vi "Live_Plot.vi"() -> ()   [LabVIEW 2013]
uses:
  <userlib>/Accelerator/User Interface/Controls/Graph.ctl
  <userlib>/Accelerator/User Interface/Controls/Constraints.ctl
  <userlib>/Accelerator/User Interface/Controls/Waveforms.ctl
  <vilib>/Utility/miscctls.llb/LVPointTypeDef.ctl
  <userlib>/_OpenG.lib/comparison/comparison.llb/Variant Changed__ogtk.vi
  <userlib>/_OpenG.lib/array/array.llb/Empty 1D Array (Variant)__ogtk.vi
panel:
  out "Multipliers":dbl[](array[numeric])
  out "Cursor grabbed?":bool
  out "Month":dbl
  out "Updating...":bool
  out "Density (g/cc)":dbl=7.874000072479248 min=0.0 max=25.0
  in  "Tab Control":T1(tab)
  out "Number of Matching Events:":i64
  out "Percent of triggers that fit constraints:":dbl format="%#_4g%"
  out "Total Number of triggers:":i64
  in  "Enable\nTimestamp":bool
  out "Constrained Distribution":T2
  in  "Save Image":bool
  in  "Constraints":T3={"Upper Timestamp Range"=timestamp(0 s since 1904-01-01), "Lower Timestamp Range"=timestamp(0 s since 1904-01-01), "Experiment Group:"="", "Experiment Name:"=[], "Upper Velocity Limit (km/s)"=0.0, "Lower Velocity Limit (km/s)"=0.0, "Upper Mass Limit (kg)"=0.0, "Lower Mass Limit (kg)"=0.0, "name array"=[], "Estimate Quality"={0.0, 5.0}} {"Estimate Quality" scale=0.0..5.0; "Lower Mass Limit (kg)" min=0.0 step=1e-20; "Upper Mass Limit (kg)" min=0.0 step=1e-20}
  in  "Velocity":dbl=1.0 min=0.1 max=100.0
  in  "Mass":dbl=2.638602750087072e-13 min=1e-20 max=1e-10
  in  "Radius (µm)":dbl=2.0 min=0.00671912 max=14.4759
  in  "Reset Visible Time":bool caption="Save Metadata"
  in  "Time Visible":dbl=5000.0 min=0.0 step=1000.0
  out "Selected Waveforms":u64[](array[numeric])
  out "Waveforms":T4[](array[typedef])
  out "Max Time":dbl=5000.0
  in  "If this was the big acc...":bool
  out "Max Query Time":dbl
  in  "Pelletron Voltage (MV):":dbl=2.0
  out "Experiment Start":timestamp
  out "Test":bool caption="Test Database in use:"
  out "Test 2":bool caption="Production Database in use:"
  in  "error in (no error)":errorcluster
  out "error out":errorcluster
  in  "Vnoise Estimate:":dbl=0.005
  in  "Sensitivity:":dbl=12100000000000.0
  in  "Update interval (s)":dbl=5.0 min=1.0 max=60.0 step=1.0 format="%#_4g"
  out "Query Time":dbl
  in  "Small?":bool
  in  "Clear Errors":bool
  in  "Exit":bool
  # "Live Plot of Current Experiment"
  # "Cursor"
  # "Plot Settings:"
  # "ODBC Connection Status:"
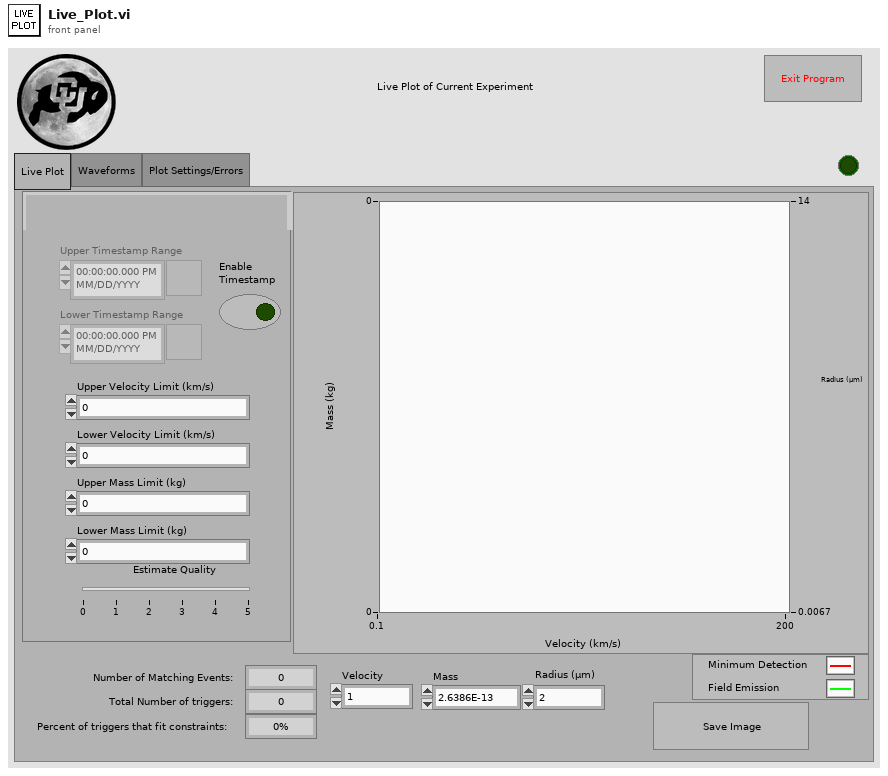
[diagram p1: front panel]
types:
  T1 = enum32{"Live Plot", "Waveforms", "Plot Settings/Errors"}
  T2 = typedef "Graph.ctl" = cluster{cluster{"Vnoise":dbl, "Vnoise":dbl}[]}[]
  T3 = typedef "Constraints.ctl" = cluster{"Upper Timestamp Range":timestamp, "Lower Timestamp Range":timestamp, "Experiment Group:":string, "Experiment Name:":i32[], "Upper Velocity Limit (km/s)":dbl, "Lower Velocity Limit (km/s)":dbl, "Upper Mass Limit (kg)":dbl, "Lower Mass Limit (kg)":dbl, "name array":string[], "Estimate Quality":cluster{dbl, dbl}}
  T4 = typedef "Waveforms.ctl" = cluster{"id_dust_event":u64, "Time Stamp":timestamp, "Velocity":dbl, "Mass":dbl, "Charge":dbl, "Radius":dbl, "Waveform Graph":sgl[][], "Quality":i32}
  T5 = typedef "LVPointTypeDef.ctl" = cluster{"Horizontal":i16, "Vertical":i16}
  T6 = typedef "LVRectTypeDef.ctl" = cluster{"Left":i16, "Top":i16, "Right":i16, "Bottom":i16}
  T7 = enum8{"Enabled", "Disabled", "Disabled and Grayed Out"}
  T8 = typedef "DisplayExperimentSetting.ctl" = cluster{"Current Experiment Name:":string, "Current Experiment Description:":string, "Current Experiment Group ID:":string, "Experiment Settings Last Updated At:":timestamp}
  T9 = typedef "Query_Dust_Event.ctl" = cluster{"Dust Event ID":i64, "Integer Timestamp":i64, "Velocity":dbl, "Mass":dbl, "Charge":sgl, "Radius":sgl, "Passed_3rd_Detector":i8, "High Voltage":sgl, "+ High Voltage Supply":sgl, "- High Voltage Supply":sgl, "HV Control Difference":sgl, "Vacuum Pressure":sgl, "Radiation":sgl, "Column Current":sgl, "Lost Charge":sgl, "Chain Current":sgl, "Control High Voltage":sgl, "Current Group Name:":string, "Current Experiment Name:":string, "Current Experiment Description:":string, "Estimate Source":T10, "Estimate Quality":i8, "File Location":T11, "Dust Type":string, "Dust Density":sgl}
  T10 = typedef "Estimate_source.ctl" = i8
  T11 = typedef "File_location.ctl" = i8
  T12 = typedef "imagedata.ctl" = cluster{"image type":i32, "image depth":i32, "image":u8[], "mask":u8[], "colors":u32[], "Rectangle":cluster{"left":i16, "top":i16, "right":i16, "bottom":i16}}
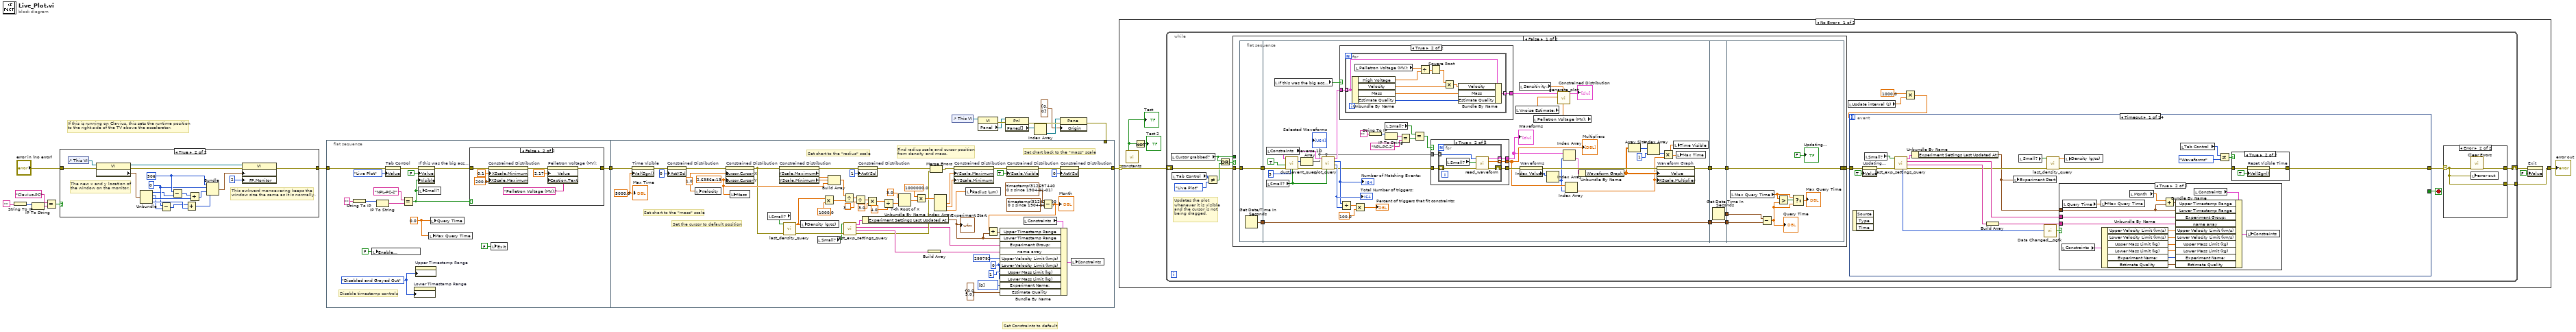
[diagram p0: block diagram]
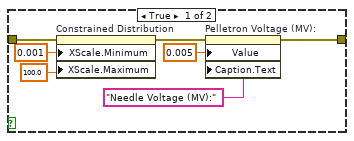
[diagram p3: hidden frame]
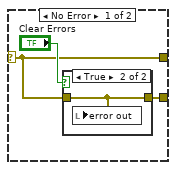
[diagram p4: hidden frame]
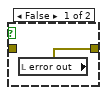
[diagram p5: hidden frame]
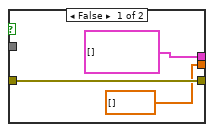
[diagram p6: hidden frame]
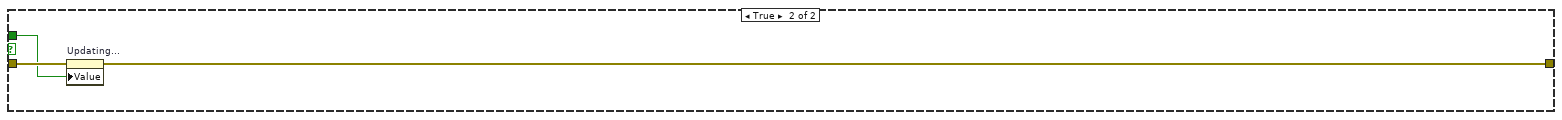
[diagram p8: hidden frame]
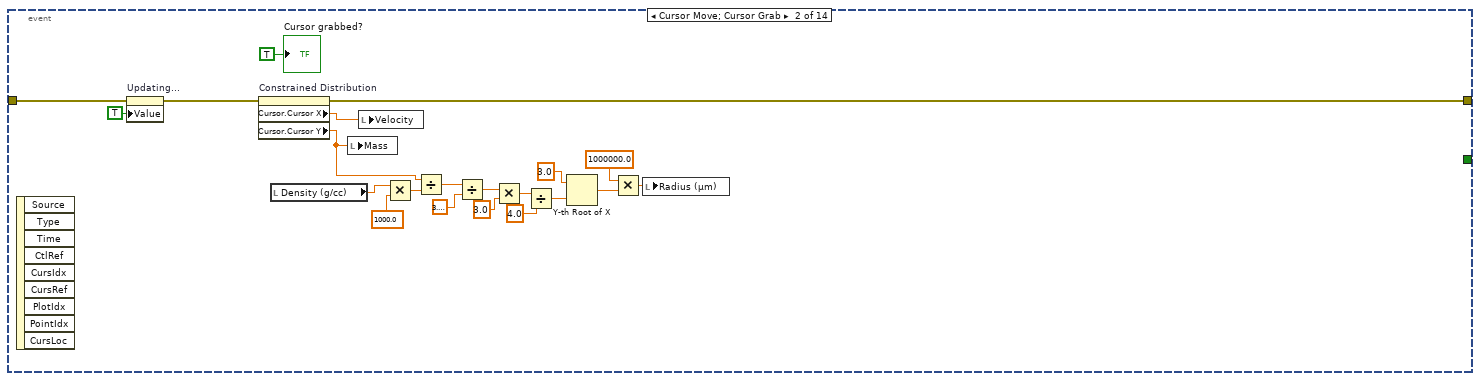
[diagram p11: hidden frame]
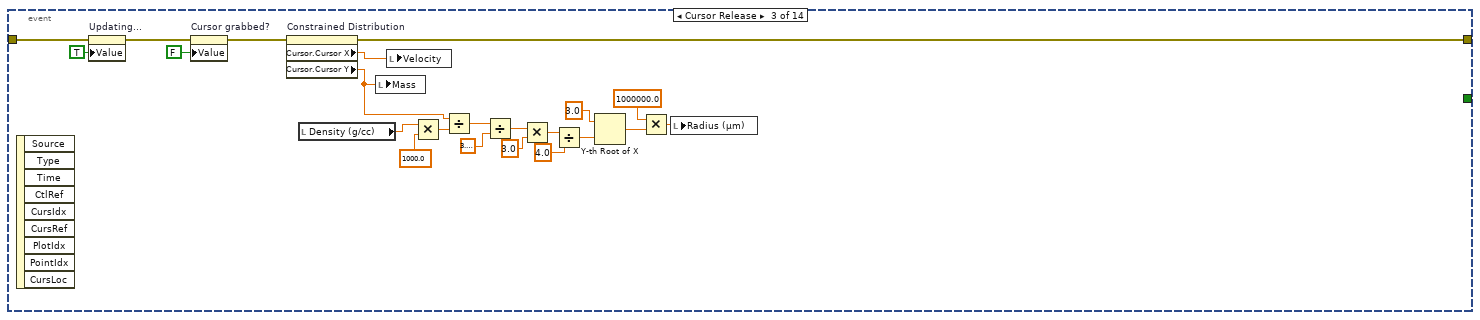
[diagram p12: hidden frame]
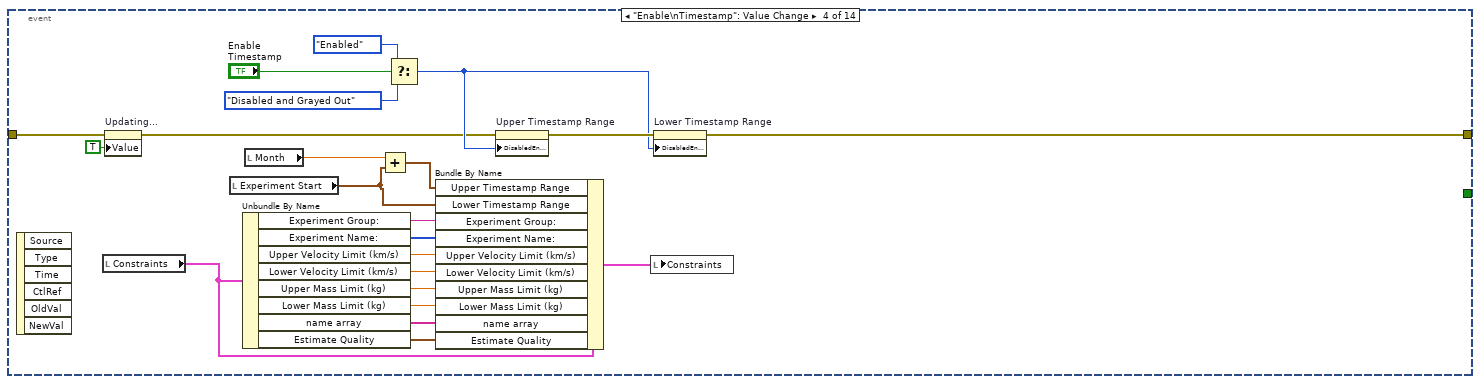
[diagram p13: hidden frame]
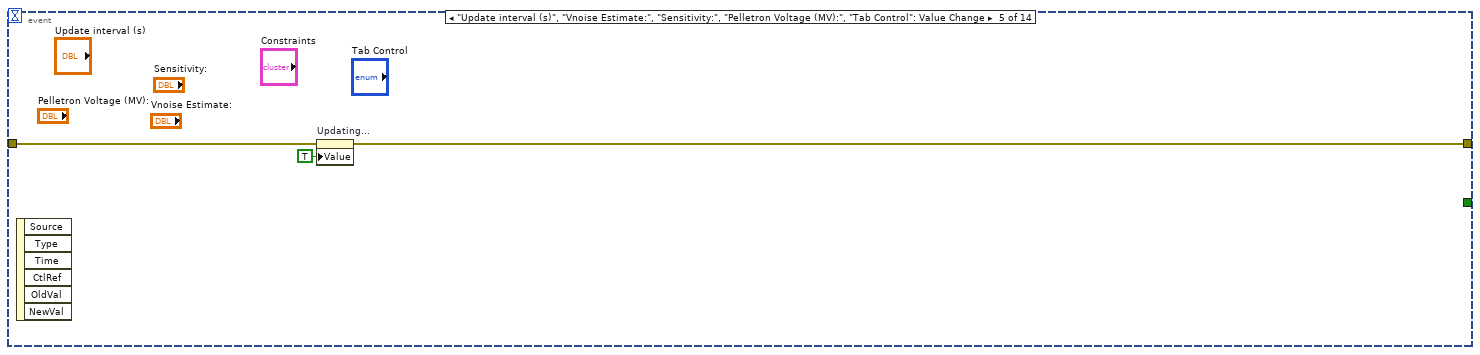
[diagram p14: hidden frame]
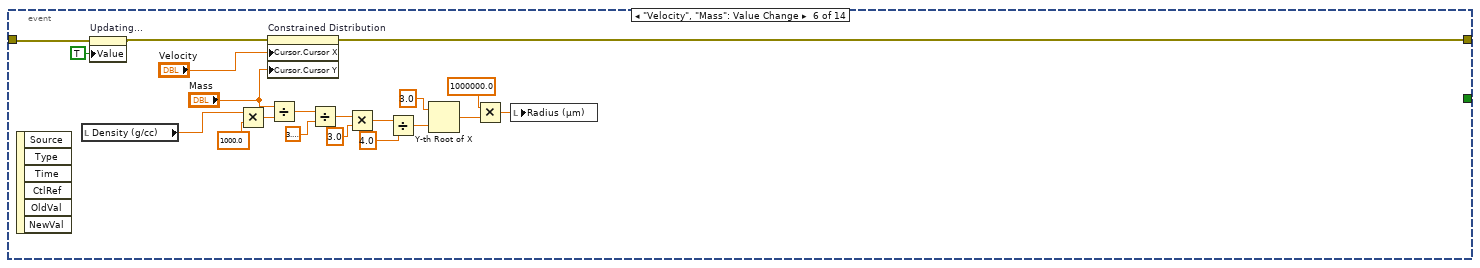
[diagram p15: hidden frame]
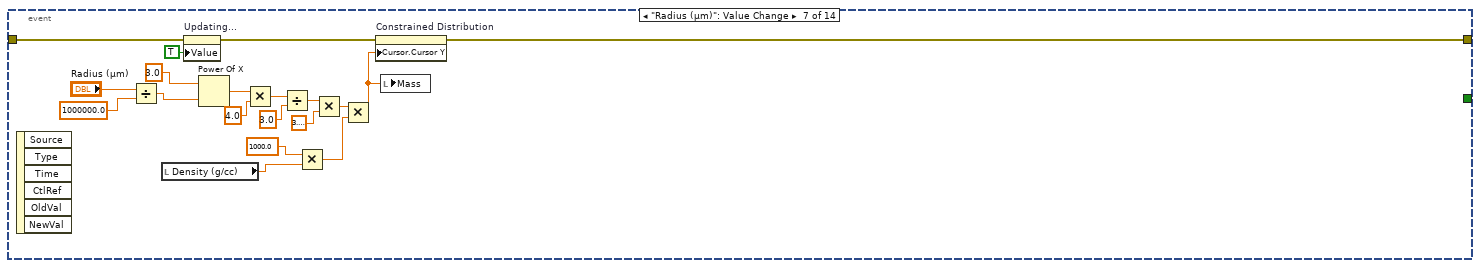
[diagram p16: hidden frame]
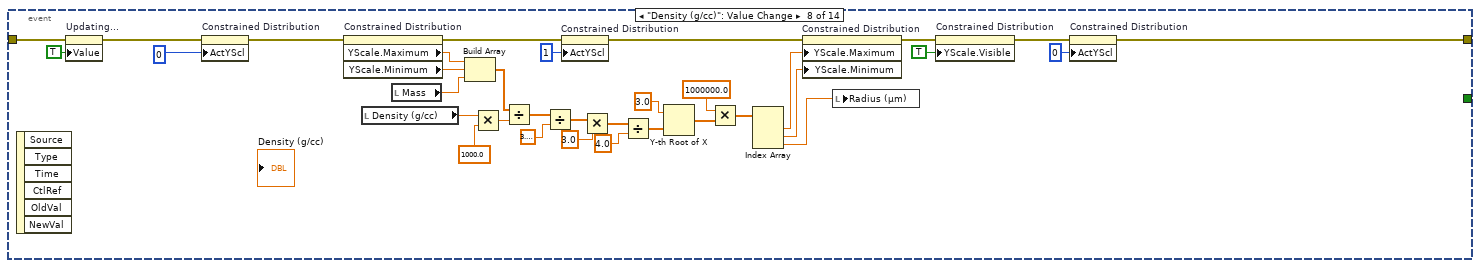
[diagram p17: hidden frame]
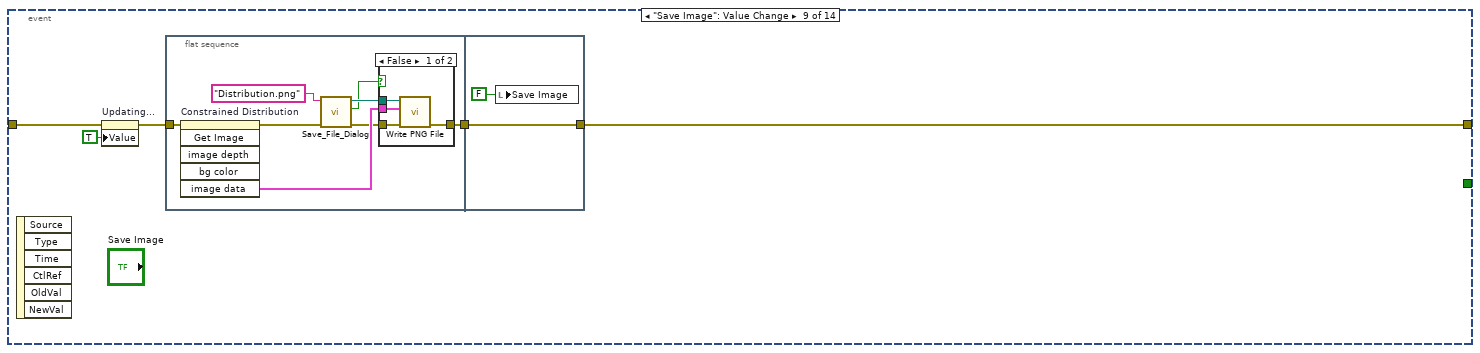
[diagram p18: hidden frame]
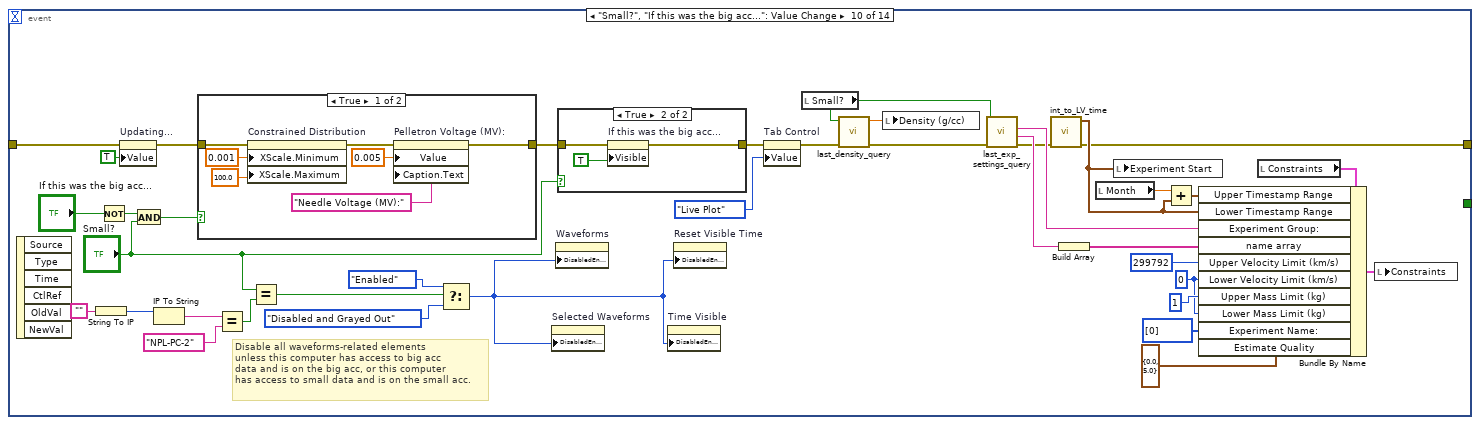
[diagram p20: hidden frame]
diagram:
  # "If this is running on Clavius, this sets the runtime position\nto the right side of the TV above the accelerator."
  # "Set Constraints to default"
  n1 = String To IP(1:"" ("name")) -> (0:w5:u32)
  n2 = IP To String(2:w5) -> (0:w3:string)  [unwired: 1 in]
  n3 = Equal?(x="Clavius-PC", y=w3) -> (x = y?=w7:bool)
  n4 = case shown="True" w7 {
    tunnel: "error in (no error)" -> [w19 w22]
    tunnel: [w19 w20] -> w1
    frame False {
    }
    frame True {
      w27 = i16 0 ("Top")
      w28 = i16 506 ("Left")
      # "This awkward manoevering keeps the\nwindow size the same as it is normally."
      # "The new x and y location of\nthe window on the monitor."
      n5 = control-ref of="This VI"() -> (w36:refnum<vi>)
      n6 = property class="VI"(reference=w36, error in=w22) -> (reference out=w32:refnum<vi>, error out=w21:errorcluster, "Front Panel.WinBounds"=w31:T6)
      n7 = Unbundle(w31) -> ("Left"=w26:i16, "Top"=w25:i16, "Right"=w30:i16, "Bottom"=w29:i16)
      n8 = Subtract(x=w27, y=w25) -> (x-y=w24:i16)
      n9 = Subtract(x=w28, y=w26) -> (x-y=w23:i16)
      n10 = Add(x=w24, y=w29) -> (x+y=w33:i16)
      n11 = Add(x=w23, y=w30) -> (x+y=w34:i16)
      n12 = Bundle("Left"=w28, "Top"=w27, w34, w33) -> (w37:cluster{"Left":i16, "Top":i16, i16, i16})  [unwired: 1 in]
      n13 = property class="VI"(reference=w32, error in=w21, "Front Panel.WinBounds"=w37, "FP.Monitor"=u16 2 ("Front Panel Window:Monitor")) -> (error out=w20:errorcluster)  [unwired: 1 out]
    }
  }
  n14 = flat-sequence {
    tunnel: [w48] -> w8
    tunnel: w1 -> [w40]
    tunnel: [w123] -> w10
    tunnel: w9 -> [_]
    tunnel: w8 -> [w73]
    frame #0 {
      w41 = 0.0 ("Query Time")
      w45 = T7."Disabled and Grayed Out" ("Disabled")
      # "Disable timestamp controls"
      n15 = String To IP(1:"" ("name")) -> (0:w51:u32)
      n16 = local write "Enable\nTimestamp"(FALSE ("Enable\nTimestamp")) -> ()
      n17 = IP To String(2:w51) -> (0:w49:string)  [unwired: 1 in]
      n18 = property on="Tab Control" class="TabCtl (strict)"(error in=w40, "Value"=T1."Live Plot" ("Tab Control")) -> (error out=w39:errorcluster)  [unwired: 1 in, 1 out]
      n19 = Equal?(x="NPL-PC-2", y=w49) -> (x = y?=w42:bool)
      n20 = property on="Lower Timestamp Range" class="AbsTime (strict)"("DisabledEnum"=w45) -> ()  [unwired: 2 in, 2 out]
      n21 = property on="Upper Timestamp Range" class="AbsTime (strict)"("DisabledEnum"=w45) -> ()  [unwired: 2 in, 2 out]
      n22 = property on="If this was the big acc..." class="Bool (strict)"(error in=w39, "Value"=FALSE ("If this was the big acc..."), "Visible"=w42) -> (error out=w44:errorcluster)  [unwired: 1 in, 1 out]
      n23 = local write "Small?"(w42) -> ()
      n24 = local write "Max Query Time"(w41) -> ()
      n25 = local write "Query Time"(w41) -> ()
      n26 = case shown="False" w42 {
        tunnel: [w57 w64] -> w48
        tunnel: w44 -> [w54 w61]
        frame True {
          n27 = property on="Constrained Distribution" class="XYGraph (strict)"(error in=w54, "XScale.Minimum"=0.001 ("X Scale.Range:Minimum"), "XScale.Maximum"=100.0 ("X Scale.Range:Maximum")) -> (error out=w53:errorcluster)  [unwired: 1 in, 1 out]
          n28 = property on="Pelletron Voltage (MV):" class="DigNum (strict)"(error in=w53, "Value"=0.005 ("Pelletron Voltage (MV):"), "Caption.Text"="Needle Voltage (MV):") -> (error out=w57:errorcluster)  [unwired: 1 in, 1 out]
        }
        frame False {
          n29 = property on="Constrained Distribution" class="XYGraph (strict)"(error in=w61, "XScale.Minimum"=0.1 ("X Scale.Range:Minimum"), "XScale.Maximum"=200.0 ("X Scale.Range:Maximum")) -> (error out=w60:errorcluster)  [unwired: 1 in, 1 out]
          n30 = property on="Pelletron Voltage (MV):" class="DigNum (strict)"(error in=w60, "Value"=2.17 ("Pelletron Voltage (MV):"), "Caption.Text"="Pelletron Voltage (MV):") -> (error out=w64:errorcluster)  [unwired: 1 in, 1 out]
        }
      }
      n31 = local write "Exit"(FALSE ("Exit")) -> ()
    }
    frame #1 {
      w71 = 5000.0 ("Max Time")
      w122 = 2.6386e-13 ("Mass")
      w109 = 1.0 ("Velocity")
      w115 = 0
      # "Set chart back to the \"mass\" scale"
      # "Set chart to the \"radius\" scale"
      # "Set chart to the \"mass\" scale"
      # "Find radius scale and cursor position\nfrom density and mass."
      # "Set the cursor to default position"
      n32 = property on="Time Visible" class="DigNum (strict)"(error in=w73, "Val(Sgnl)"=w71) -> (error out=w72:errorcluster)  [unwired: 1 in, 1 out]
      n33 = property on="Constrained Distribution" class="XYGraph (strict)"(error in=w72, "ActYScl"=0 ("Active Y Scale")) -> (error out=w78:errorcluster)  [unwired: 1 in, 1 out]
      n34 = local write "Velocity"(w109) -> ()
      n35 = property on="Constrained Distribution" class="XYGraph (strict)"(error in=w78, "Cursor.Cursor X"=w109, "Cursor.Cursor Y"=w122) -> (error out=w80:errorcluster)  [unwired: 1 in, 1 out]
      n36 = local write "Mass"(w122) -> ()
      n37 = local read "Small?"() -> (w77:bool)
      n38 = property on="Constrained Distribution" class="XYGraph (strict)"(error in=w80) -> (error out=w96:errorcluster, "YScale.Maximum"=w95:dbl, "YScale.Minimum"=w94:dbl)  [unwired: 1 in, 1 out]
      n39 = call <userlib>:"last_density_query.vi"("error in (no error)"=w80, "Small?"=w77) -> ("error out"=w82:errorcluster, "Density"=w81:dbl)  [unwired: 8 in]
      n40 = local write "Density (g/cc)"(w81) -> ()
      n41 = local read "Small?"() -> (w76:bool)
      n42 = Multiply(x=w81, y=1000.0) -> (x*y=w100:dbl)
      n43 = Build Array(w95, w94, w122) -> (w93:dbl[])
      n44 = Divide(x=w93, y=w100) -> (x/y=w108:dbl[])
      n45 = call <userlib>:"last_exp_settings_query.vi"("error in (no error)"=w82, "Small?"=w76) -> ("error out"=w70:errorcluster, "Experiment Name"=w110:string, "Group Name"=w67:string, "Experiment Settings"=w69:T8)  [unwired: 4 in, 2 out]
      n46 = Divide(x=w108, y=3.141592653589793) -> (x/y=w106:dbl[])
      n47 = property on="Constrained Distribution" class="XYGraph (strict)"(error in=w96, "ActYScl"=1 ("Active Y Scale")) -> (error out=w92:errorcluster)  [unwired: 1 in, 1 out]
      n48 = Unbundle By Name(w69) -> ("Experiment Settings Last Updated At:"=w68:timestamp)
      "Experiment Start" <- w68
      n49 = Multiply(x=w106, y=3.0) -> (x*y=w104:dbl[])
      n50 = Divide(x=w104, y=4.0) -> (x/y=w102:dbl[])
      n51 = Y-th Root of X(1:w102, 2:3.0 ("y")) -> (0:w98:dbl[])
      n52 = Multiply(x=1000000.0, y=w98) -> (x*y=w90:dbl[])
      n53 = Build Array(w110) -> (w74:string[])
      n54 = Merge Errors(w92, w70) -> (w75:errorcluster)
      n55 = Index Array(array=w90) -> (element #1=w88:dbl, element #2=w87:dbl, element #3=w86:dbl)  [unwired: 3 in]
      n56 = property on="Constrained Distribution" class="XYGraph (strict)"(error in=w75, "YScale.Maximum"=w88, "YScale.Minimum"=w87) -> (error out=w89:errorcluster)  [unwired: 1 in, 1 out]
      n57 = local write "Radius (µm)"(w86) -> ()
      n58 = property on="Constrained Distribution" class="XYGraph (strict)"(error in=w89, "YScale.Visible"=TRUE ("Y Scale.Visible")) -> (error out=w84:errorcluster)  [unwired: 1 in, 1 out]
      n59 = local read "Constraints"() -> (w121:T3)
      n60 = Subtract(x=timestamp(3126974400 s since 1904-01-01) ("current time"), y=timestamp(3124296000 s since 1904-01-01) ("current time")) -> (x-y=w118:dbl)
      "Month" <- w118
      n61 = Add(x=w118, y=w68) -> (x+y=w119:timestamp)
      n62 = Bundle By Name(cluster=w121, "Upper Timestamp Range"=w119, "Lower Timestamp Range"=w68, "Experiment Group:"=w67, "name array"=w74, "Upper Velocity Limit (km/s)"=299792, "Lower Velocity Limit (km/s)"=w115, "Upper Mass Limit (kg)"=1, "Lower Mass Limit (kg)"=w115, "Experiment Name:"=i32[] [0], "Estimate Quality"=cluster{dbl, dbl} {0.0, 5.0}) -> (w120:T3)
      n63 = property on="Constrained Distribution" class="XYGraph (strict)"(error in=w84, "ActYScl"=0 ("Active Y Scale")) -> (error out=w123:errorcluster)  [unwired: 1 in, 1 out]
      n64 = local write "Constraints"(w120) -> ()
      "Max Time" <- w71
    }
  }
  n65 = control-ref of="This VI"() -> (w17:refnum<vi>)
  n66 = property class="VI"(reference=w17) -> (error out=w16:errorcluster, "Panel"=w15:refnum<vi>)  [unwired: 1 in, 1 out]
  n67 = property class="Pnl"(reference=w15, error in=w16) -> (error out=w14:errorcluster, "Panes[]"=w13:refnum<vi>[])  [unwired: 1 out]
  n68 = Index Array(array=w13) -> (element=w12:refnum<vi>)  [unwired: 1 in]
  n69 = property class="Pane"(reference=w12, error in=w14, "Origin"=T5 {"Horizontal"=0, "Vertical"=0}) -> (error out=w9:errorcluster)  [unwired: 1 out]
  n70 = case shown="No Error" w10 {
    selector: w10 -> [w125 w560]
    tunnel: [w128 w560] -> w18
    frame No Error {
      n71 = call <userlib>:"constants.vi"() -> ("Testing"=w124:bool)  [unwired: 3 out]
      "Test" <- w124
      n72 = Not(x=w124) -> (.not. x?=→"Test 2":bool)
      n73 = while {
        shift-right: [w131] -> w127
        shift-left: w125 -> [w139]
        tunnel: [w130] -> w128
        stop <- w141 stop-if-true
        # "Updates the plot\nwhenever it is visible\nand the cursor is not\nbeing dragged."
        n74 = local read "Cursor grabbed?"() -> (w133:bool)
        n75 = local read "Tab Control"() -> (w137:T1)
        n76 = Not Equal?(x=w137, y=T1."Live Plot") -> (x != y?=w135:bool)
        n77 = Or(x=w133, y=w135) -> (x .or. y?=w136:bool)
        n78 = case shown="False" w136 {
          tunnel: [w152 w243] -> w140
          tunnel: w139 -> [w151 w245]
          tunnel: w133 -> [_ w244]
          frame False {
            n79 = flat-sequence {
              tunnel: w151 -> [w161]
              tunnel: [w161] -> w159
              tunnel: [w160] -> w158
              tunnel: w159 -> [w191]
              tunnel: [w173] -> w157
              tunnel: [w196] -> w156
              tunnel: w158 -> [w196]
              tunnel: w157 -> [w234]
              tunnel: [w234] -> w155
              tunnel: w156 -> [w233]
              tunnel: [w233] -> w154
              tunnel: [w232] -> w153
              tunnel: [w242] -> w152
              tunnel: w155 -> [w242]
              tunnel: w154 -> [w241]
              tunnel: w153 -> [w236]
              frame #0 {
                n80 = Get Date/Time In Seconds() -> (seconds since 1Jan1904=w160:timestamp)
              }
              frame #1 {
                n81 = local read "Constraints"() -> (w189:T3)
                n82 = local read "Small?"() -> (w180:bool)
                n83 = local read "If this was the big acc..."() -> (w192:bool)
                n84 = call <userlib>:"dust_event_query.vi"("No. of Events"=u64 5 ("Limit no. of events"), "error in (no error)"=w191, "Limited?"=TRUE, "Small?"=w180, "Constraints"=w189) -> ("error out"=w190:errorcluster, "Dust Event ID Array"=w178:i64[])  [unwired: 2 in, 3 out]
                n85 = Reverse 1D Array(array=w178) -> (reversed array=w177:i64[])
                "Selected Waveforms" <- w177
                n86 = call <userlib>:"plot_query.vi"("Small?"=w180, "Selected Dust Events"=w177, "error in (no error)"=w190, "Constraints"=w189) -> ("error out"=w186:errorcluster, "Total Number of triggers"=w197:u64, "Number of Matching Events"=w195:u64, "Dust Array"=w194:T9[])  [unwired: 3 in, 1 out]
                "Total Number of triggers:" <- w197
                "Number of Matching Events:" <- w195
                n87 = case shown="True" w192 {
                  tunnel: w194 -> [w219 w221]
                  tunnel: [w219 w220] -> w193
                  frame False {
                  }
                  frame True {
                    n88 = for {
                      tunnel: w221 -> [w231] mode=indexing
                      tunnel: [w230] -> w220 mode=indexing
                      n89 = Unbundle By Name(w231) -> ("High Voltage"=w226:sgl, "Velocity"=w225:dbl, "Mass"=w228:dbl, "Estimate Quality"=w229:i8)
                      n90 = local read "Pelletron Voltage (MV):"() -> (w227:dbl)
                      n91 = Divide(x=w227, y=w226) -> (x/y=w223:dbl)
                      n92 = Square Root(x=w223) -> (sqrt(x)=w222:dbl)
                      n93 = Multiply(x=w222, y=w225) -> (x*y=w224:dbl)
                      n94 = Bundle By Name(cluster=w231, "Velocity"=w224, "Mass"=w228, "Estimate Quality"=w229) -> (w230:T9)
                    }
                  }
                }
                n95 = Divide(x=w195, y=w197) -> (x/y=w200:dbl)
                n96 = Multiply(x=w200, y=100.0) -> (x*y=→"Percent of triggers that fit constraints:":dbl)
                n97 = String To IP(1:"" ("name")) -> (0:w183:u32)
                n98 = IP To String(2:w183) -> (0:w181:string)  [unwired: 1 in]
                n99 = local read "Small?"() -> (w176:bool)
                n100 = Equal?(x=w181, y="NPL-PC-2" ("x")) -> (x = y?=w185:bool)
                n101 = Equal?(x=w176, y=w185) -> (x = y?=w179:bool)
                n102 = case shown="True" w179 {
                  tunnel: w186 -> [w206 w212]
                  tunnel: [T4[] [] ("Waveforms") w211] -> w170
                  tunnel: [w206 w210] -> w175
                  tunnel: w177 -> [_ w209]
                  tunnel: [dbl[] [] w208] -> w171
                  frame False {
                  }
                  frame True {
                    n103 = for {
                      tunnel: [w216] -> w211 mode=indexing
                      shift-right: [w215] -> w210
                      shift-left: w212 -> [w217]
                      tunnel: w209 -> [w214] mode=indexing
                      tunnel: [w213] -> w208 mode=indexing
                      n104 = local read "Small?"() -> (w218:bool)
                      n105 = call <userlib>:"read_waveform.vi"("error in (no error)"=w217, "Small?"=w218, "Dust Event ID"=w214) -> ("error out"=w215:errorcluster, "multiplier"=w213:dbl, "Waveform"=w216:T4)  [unwired: 6 in]
                    }
                  }
                }
                "Waveforms" <- w170
                "Multipliers" <- w171
                n106 = local read "Vnoise Estimate:"() -> (w202:dbl)
                n107 = local read "Sensitivity:"() -> (w203:dbl)
                n108 = property on="Waveforms" class="Arr (strict)"(error in=w175) -> (error out=w174:errorcluster, "Index Values"=w172:u32[])  [unwired: 1 in, 1 out]
                n109 = local read "Pelletron Voltage (MV):"() -> (w201:dbl)
                n110 = Index Array(array=w172) -> (element=w169:u32)  [unwired: 1 in]
                n111 = call <userlib>:"generate_plot.vi"("High Voltage"=w201, "Sens"=w203, "Vnoise"=w202, "Dust Array"=w193) -> ("Dust Distribution"=→"Constrained Distribution":T2)  [unwired: 7 in]
                n112 = Index Array(array=w170, index=w169) -> (element=w168:T4)
                n113 = Index Array(array=w171, index=w169) -> (element=w163:dbl)
                n114 = Unbundle By Name(w168) -> ("Waveform Graph"=w164:sgl[][])
                n115 = Array Size(array=w164) -> (size(s)=w165:i32[])
                n116 = Index Array(array=w165, index=1) -> (element=w167:i32)
                n117 = property on="Waveform Graph" class="WFGraph (strict)"(error in=w174, "Value"=w164, "XScale.Multiplier"=w163) -> (error out=w173:errorcluster)  [unwired: 1 in, 1 out]
                n118 = Multiply(x=w167, y=w163) -> (x*y=w162:dbl)
                n119 = local write "Time Visible"(w162) -> ()
                n120 = local write "Max Time"(w162) -> ()
              }
              frame #2 {
                n121 = Get Date/Time In Seconds() -> (seconds since 1Jan1904=w232:timestamp)
              }
              frame #3 {
                n122 = local read "Max Query Time"() -> (w239:dbl)
                n123 = Subtract(x=w236, y=w241) -> (x-y=w238:dbl)
                "Query Time" <- w238
                n124 = Greater?(x=w239, y=w238) -> (0:w240:bool)
                n125 = Select(t=w239, s=w240, f=w238) -> (s? t:f=→"Max Query Time":dbl)
                "Updating..." <- FALSE ("Updating...")
              }
            }
          }
          frame True {
            n126 = property on="Updating..." class="Bool (strict)"(error in=w245, "Value"=w244) -> (error out=w243:errorcluster)  [unwired: 1 in, 1 out]
          }
        }
        n127 = local read "Update interval (s)"() -> (w138:dbl)
        n128 = Multiply(x=1000.0, y=w138) -> (x*y=w142:dbl)
        n129 = event shown="[0] Timeout" {
          selector: _ -> [_ _ _ _ _ _ _ _ _ _ _ _ _ _]
          dyn-events: _ -> [_ _ _ _ _ _ _ _ _ _ _ _ _ _]
          timeout: w142 -> [_ _ _ _ _ _ _ _ _ _ _ _ _ _]
          tunnel: w140 -> [w257 w284 w306 w328 w351 w352 w372 w393 w425 w458 w516 w535 w545 w559]
          tunnel: [w255 w288 w308 w335 w350 w371 w390 w397 w429 w466 w519 w537 w541 w559] -> w132
          tunnel: [_ _ _ _ _ _ _ _ _ _ _ _ _ "Exit"] -> w141
          event Timeout {
            n130 = event-data() -> ()  [unwired: 1 in, 3 out]
            n131 = property on="Updating..." class="Bool (strict)"(error in=w257, "Value"=TRUE ("Updating...")) -> (error out=w258:errorcluster)  [unwired: 1 in, 1 out]
            n132 = local read "Small?"() -> (w261:bool)
            n133 = call <userlib>:"last_exp_settings_query.vi"("error in (no error)"=w258, "Small?"=w261) -> ("error out"=w249:errorcluster, "Experiment Name"=w264:string, "Group Name"=w263:string, "Experiment Settings"=w248:T8, "Experiment ID"=w250:i64)  [unwired: 4 in, 1 out]
            n134 = Unbundle By Name(w248) -> ("Experiment Settings Last Updated At:"=w247:timestamp)
            n135 = Build Array(w264) -> (w251:string[])
            n136 = local write "Experiment Start"(w247) -> ()
            n137 = local read "Small?"() -> (w260:bool)
            n138 = call-poly <userlib>:"Data Changed__ogtk.vi"("Variant"=w250) -> ("Changed"=w246:bool)
            n139 = call <userlib>:"last_density_query.vi"("error in (no error)"=w249, "Small?"=w260) -> ("error out"=w256:errorcluster, "Density"=w262:dbl)  [unwired: 8 in]
            n140 = case shown="True" w246 {
              tunnel: w263 -> [_ w276]
              tunnel: w247 -> [_ w267]
              tunnel: w251 -> [_ w266]
              frame False {
              }
              frame True {
                n141 = local read "Constraints"() -> (w274:T3)
                n142 = local read "Query Time"() -> (w265:dbl)
                n143 = local write "Max Query Time"(w265) -> ()
                n144 = Unbundle By Name(w274) -> ("Upper Velocity Limit (km/s)"=w273:dbl, "Lower Velocity Limit (km/s)"=w272:dbl, "Upper Mass Limit (kg)"=w271:dbl, "Lower Mass Limit (kg)"=w270:dbl, "Experiment Name:"=w269:i32[], "Estimate Quality"=w268:cluster{dbl, dbl})
                n145 = local read "Month"() -> (w275:dbl)
                n146 = Add(x=w275, y=w267) -> (x+y=w277:timestamp)
                n147 = local read "Constraints"() -> (w279:T3)
                n148 = Bundle By Name(cluster=w279, "Upper Timestamp Range"=w277, "Lower Timestamp Range"=w267, "Experiment Group:"=w276, "name array"=w266, "Upper Velocity Limit (km/s)"=w273, "Lower Velocity Limit (km/s)"=w272, "Upper Mass Limit (kg)"=w271, "Lower Mass Limit (kg)"=w270, "Experiment Name:"=w269, "Estimate Quality"=w268) -> (w278:T3)
                n149 = local write "Constraints"(w278) -> ()
              }
            }
            n150 = local write "Density (g/cc)"(w262) -> ()
            n151 = local read "Tab Control"() -> (w253:T1)
            n152 = Not Equal?(x=w253, y=T1."Waveforms") -> (x != y?=w254:bool)
            n153 = case shown="True" w254 {
              tunnel: w256 -> [w280 w283]
              tunnel: [w280 w282] -> w255
              frame False {
              }
              frame True {
                n154 = property on="Reset Visible Time" class="Bool (strict)"(error in=w283, "Val(Sgnl)"=TRUE ("Value (Signaling)")) -> (error out=w282:errorcluster)  [unwired: 1 in, 1 out]
              }
            }
          }
          event Cursor Move; Cursor Grab {
            n155 = event-data() -> ()  [unwired: 1 in, 9 out]
            n156 = property on="Updating..." class="Bool (strict)"(error in=w284, "Value"=TRUE ("Updating...")) -> (error out=w285:errorcluster)  [unwired: 1 in, 1 out]
            n157 = property on="Constrained Distribution" class="XYGraph (strict)"(error in=w285) -> (error out=w288:errorcluster, "Cursor.Cursor X"=w304:dbl, "Cursor.Cursor Y"=w291:dbl)  [unwired: 1 in, 1 out]
            n158 = local read "Density (g/cc)"() -> (w290:dbl)
            n159 = local write "Mass"(w291) -> ()
            n160 = local write "Velocity"(w304) -> ()
            n161 = Multiply(x=w290, y=1000.0) -> (x*y=w295:dbl)
            n162 = Divide(x=w291, y=w295) -> (x/y=w303:dbl)
            n163 = Divide(x=w303, y=3.141592653589793) -> (x/y=w301:dbl)
            n164 = Multiply(x=w301, y=3.0) -> (x*y=w299:dbl)
            n165 = Divide(x=w299, y=4.0) -> (x/y=w297:dbl)
            n166 = Y-th Root of X(1:w297, 2:3.0 ("y")) -> (0:w293:dbl)
            n167 = Multiply(x=1000000.0, y=w293) -> (x*y=w289:dbl)
            n168 = local write "Radius (µm)"(w289) -> ()
            "Cursor grabbed?" <- TRUE ("Updating...")
          }
          event Cursor Release {
            n169 = event-data() -> ()  [unwired: 1 in, 9 out]
            n170 = property on="Updating..." class="Bool (strict)"(error in=w306, "Value"=TRUE ("Updating...")) -> (error out=w305:errorcluster)  [unwired: 1 in, 1 out]
            n171 = property on="Cursor grabbed?" class="Bool (strict)"(error in=w305, "Value"=FALSE ("Cursor grabbed?")) -> (error out=w309:errorcluster)  [unwired: 1 in, 1 out]
            n172 = property on="Constrained Distribution" class="XYGraph (strict)"(error in=w309) -> (error out=w308:errorcluster, "Cursor.Cursor X"=w325:dbl, "Cursor.Cursor Y"=w312:dbl)  [unwired: 1 in, 1 out]
            n173 = local read "Density (g/cc)"() -> (w311:dbl)
            n174 = local write "Mass"(w312) -> ()
            n175 = local write "Velocity"(w325) -> ()
            n176 = Multiply(x=w311, y=1000.0) -> (x*y=w316:dbl)
            n177 = Divide(x=w312, y=w316) -> (x/y=w324:dbl)
            n178 = Divide(x=w324, y=3.141592653589793) -> (x/y=w322:dbl)
            n179 = Multiply(x=w322, y=3.0) -> (x*y=w320:dbl)
            n180 = Divide(x=w320, y=4.0) -> (x/y=w318:dbl)
            n181 = Y-th Root of X(1:w318, 2:3.0 ("y")) -> (0:w314:dbl)
            n182 = Multiply(x=1000000.0, y=w314) -> (x*y=w310:dbl)
            n183 = local write "Radius (µm)"(w310) -> ()
          }
          event "Enable\nTimestamp": Value Change {
            n184 = event-data() -> ()  [unwired: 1 in, 6 out]
            n185 = local read "Constraints"() -> (w348:T3)
            n186 = property on="Updating..." class="Bool (strict)"(error in=w328, "Value"=TRUE ("Updating...")) -> (error out=w329:errorcluster)  [unwired: 1 in, 1 out]
            n187 = local read "Experiment Start"() -> (w330:timestamp)
            n188 = Unbundle By Name(w348) -> ("Experiment Group:"=w339:string, "Experiment Name:"=w340:i32[], "Upper Velocity Limit (km/s)"=w341:dbl, "Lower Velocity Limit (km/s)"=w342:dbl, "Upper Mass Limit (kg)"=w343:dbl, "Lower Mass Limit (kg)"=w344:dbl, "name array"=w345:string[], "Estimate Quality"=w346:cluster{dbl, dbl})
            n189 = local read "Month"() -> (w337:dbl)
            n190 = Add(x=w337, y=w330) -> (x+y=w338:timestamp)
            n191 = Select(t=T7."Enabled" ("Disabled"), s="Enable\nTimestamp", f=T7."Disabled and Grayed Out" ("Disabled")) -> (s? t:f=w331:T7)
            n192 = Bundle By Name(cluster=w348, "Upper Timestamp Range"=w338, "Lower Timestamp Range"=w330, "Experiment Group:"=w339, "Experiment Name:"=w340, "Upper Velocity Limit (km/s)"=w341, "Lower Velocity Limit (km/s)"=w342, "Upper Mass Limit (kg)"=w343, "Lower Mass Limit (kg)"=w344, "name array"=w345, "Estimate Quality"=w346) -> (w347:T3)
            n193 = property on="Upper Timestamp Range" class="AbsTime (strict)"(error in=w329, "DisabledEnum"=w331) -> (error out=w336:errorcluster)  [unwired: 1 in, 1 out]
            n194 = local write "Constraints"(w347) -> ()
            n195 = property on="Lower Timestamp Range" class="AbsTime (strict)"(error in=w336, "DisabledEnum"=w331) -> (error out=w335:errorcluster)  [unwired: 1 in, 1 out]
          }
          event "Update interval (s)", "Vnoise Estimate:", "Sensitivity:", "Pelletron Voltage (MV):", "Tab Control": Value Change {
            n196 = event-data() -> ()  [unwired: 1 in, 6 out]
            n197 = property on="Updating..." class="Bool (strict)"(error in=w351, "Value"=TRUE ("Updating...")) -> (error out=w350:errorcluster)  [unwired: 1 in, 1 out]
          }
          event "Velocity", "Mass": Value Change {
            n198 = event-data() -> ()  [unwired: 1 in, 6 out]
            n199 = local read "Density (g/cc)"() -> (w369:dbl)
            n200 = property on="Updating..." class="Bool (strict)"(error in=w352, "Value"=TRUE ("Updating...")) -> (error out=w353:errorcluster)  [unwired: 1 in, 1 out]
            n201 = Multiply(x=w369, y=1000.0) -> (x*y=w360:dbl)
            n202 = property on="Constrained Distribution" class="XYGraph (strict)"(error in=w353, "Cursor.Cursor X"="Velocity", "Cursor.Cursor Y"="Mass") -> (error out=w371:errorcluster)  [unwired: 1 in, 1 out]
            n203 = Divide(x="Mass", y=w360) -> (x/y=w368:dbl)
            n204 = Divide(x=w368, y=3.141592653589793) -> (x/y=w366:dbl)
            n205 = Multiply(x=w366, y=3.0) -> (x*y=w364:dbl)
            n206 = Divide(x=w364, y=4.0) -> (x/y=w362:dbl)
            n207 = Y-th Root of X(1:w362, 2:3.0 ("y")) -> (0:w357:dbl)
            n208 = Multiply(x=1000000.0, y=w357) -> (x*y=w356:dbl)
            n209 = local write "Radius (µm)"(w356) -> ()
          }
          event "Radius (µm)": Value Change {
            n210 = event-data() -> ()  [unwired: 1 in, 6 out]
            n211 = Divide(x="Radius (µm)", y=1000000.0) -> (x/y=w381:dbl)
            n212 = local read "Density (g/cc)"() -> (w375:dbl)
            n213 = property on="Updating..." class="Bool (strict)"(error in=w372, "Value"=TRUE ("Updating...")) -> (error out=w373:errorcluster)  [unwired: 1 in, 1 out]
            n214 = Power Of X(1:w381, 2:3.0 ("y")) -> (0:w380:dbl)
            n215 = Multiply(x=w380, y=4.0) -> (x*y=w387:dbl)
            n216 = Divide(x=w387, y=3.0) -> (x/y=w385:dbl)
            n217 = Multiply(x=1000.0, y=w375) -> (x*y=w378:dbl)
            n218 = Multiply(x=w385, y=3.141592653589793) -> (x*y=w379:dbl)
            n219 = Multiply(x=w379, y=w378) -> (x*y=w376:dbl)
            n220 = property on="Constrained Distribution" class="XYGraph (strict)"(error in=w373, "Cursor.Cursor Y"=w376) -> (error out=w390:errorcluster)  [unwired: 1 in, 1 out]
            n221 = local write "Mass"(w376) -> ()
          }
          event "Density (g/cc)": Value Change {
            n222 = event-data() -> ()  [unwired: 1 in, 6 out]
            n223 = property on="Updating..." class="Bool (strict)"(error in=w393, "Value"=TRUE ("Updating...")) -> (error out=w391:errorcluster)  [unwired: 1 in, 1 out]
            n224 = property on="Constrained Distribution" class="XYGraph (strict)"(error in=w391, "ActYScl"=0 ("Active Y Scale")) -> (error out=w409:errorcluster)  [unwired: 1 in, 1 out]
            n225 = property on="Constrained Distribution" class="XYGraph (strict)"(error in=w409) -> (error out=w411:errorcluster, "YScale.Maximum"=w412:dbl, "YScale.Minimum"=w413:dbl)  [unwired: 1 in, 1 out]
            n226 = local read "Density (g/cc)"() -> (w407:dbl)
            n227 = local read "Mass"() -> (w398:dbl)
            n228 = Build Array(w412, w413, w398) -> (w414:dbl[])
            n229 = Multiply(x=w407, y=1000.0) -> (x*y=w405:dbl)
            n230 = Divide(x=w414, y=w405) -> (x/y=w399:dbl[])
            n231 = Divide(x=w399, y=3.141592653589793) -> (x/y=w401:dbl[])
            n232 = property on="Constrained Distribution" class="XYGraph (strict)"(error in=w411, "ActYScl"=1 ("Active Y Scale")) -> (error out=w415:errorcluster)  [unwired: 1 in, 1 out]
            n233 = Multiply(x=w401, y=3.0) -> (x*y=w402:dbl[])
            n234 = Divide(x=w402, y=4.0) -> (x/y=w403:dbl[])
            n235 = Y-th Root of X(1:w403, 2:3.0 ("y")) -> (0:w406:dbl[])
            n236 = Multiply(x=1000000.0, y=w406) -> (x*y=w417:dbl[])
            n237 = Index Array(array=w417) -> (element #1=w419:dbl, element #2=w420:dbl, element #3=w421:dbl)  [unwired: 3 in]
            n238 = property on="Constrained Distribution" class="XYGraph (strict)"(error in=w415, "YScale.Maximum"=w419, "YScale.Minimum"=w420) -> (error out=w418:errorcluster)  [unwired: 1 in, 1 out]
            n239 = local write "Radius (µm)"(w421) -> ()
            n240 = property on="Constrained Distribution" class="XYGraph (strict)"(error in=w418, "YScale.Visible"=TRUE ("Y Scale.Visible")) -> (error out=w423:errorcluster)  [unwired: 1 in, 1 out]
            n241 = property on="Constrained Distribution" class="XYGraph (strict)"(error in=w423, "ActYScl"=0 ("Active Y Scale")) -> (error out=w397:errorcluster)  [unwired: 1 in, 1 out]
          }
          event "Save Image": Value Change {
            n242 = event-data() -> ()  [unwired: 1 in, 6 out]
            n243 = property on="Updating..." class="Bool (strict)"(error in=w425, "Value"=TRUE ("Updating...")) -> (error out=w426:errorcluster)  [unwired: 1 in, 1 out]
            n244 = flat-sequence {
              tunnel: [w436] -> w428
              tunnel: w426 -> [w435]
              tunnel: [w444] -> w429
              tunnel: w428 -> [w444]
              frame #0 {
                n245 = invoke on="Constrained Distribution" class="XYGraph (strict)" method="Get Image"(error in=w435) -> (error out=w434:errorcluster, "image data"=w437:T12)  [unwired: 5 in, 4 out]
                n246 = call <userlib>:"Save_File_Dialog.vi"("error in (no error)"=w434, "Filename"="Distribution.png") -> ("error out"=w432:errorcluster, "Cancelled"=w430:bool, "Path"=w431:path)  [unwired: 7 in]
                n247 = case shown="False" w430 {
                  tunnel: w437 -> [w441 _]
                  tunnel: [w440 w442] -> w436
                  tunnel: w431 -> [w439 _]
                  tunnel: w432 -> [w438 w442]
                  frame False {
                    n248 = call <vilib>:"Write PNG File.vi"("error in (no error)"=w438, "image data"=w441, "path to PNG file"=w439) -> ("error out"=w440:errorcluster)  [unwired: 7 in, 1 out]
                  }
                  frame True {
                  }
                }
              }
              frame #1 {
                n249 = local write "Save Image"(FALSE ("Save Image")) -> ()
              }
            }
          }
          event "Small?", "If this was the big acc...": Value Change {
            w475 = 0
            # "Disable all waveforms-related elements\nunless this computer has access to big acc\ndata and is on the big acc, or this computer\nhas access to small data and is on the small acc."
            n250 = event-data() -> ()  [unwired: 1 in, 6 out]
            n251 = String To IP(1:"" ("name")) -> (0:w453:u32)
            n252 = Not(x="If this was the big acc...") -> (.not. x?=w463:bool)
            n253 = property on="Updating..." class="Bool (strict)"(error in=w458, "Value"=TRUE ("Updating...")) -> (error out=w457:errorcluster)  [unwired: 1 in, 1 out]
            n254 = And(x=w463, y="Small?") -> (x .and. y?=w465:bool)
            n255 = IP To String(2:w453) -> (0:w455:string)  [unwired: 1 in]
            n256 = case shown="True" w465 {
              tunnel: [w493 w500] -> w462
              tunnel: w457 -> [w490 w497]
              frame True {
                n257 = property on="Constrained Distribution" class="XYGraph (strict)"(error in=w490, "XScale.Minimum"=0.001 ("X Scale.Range:Minimum"), "XScale.Maximum"=100.0 ("X Scale.Range:Maximum")) -> (error out=w489:errorcluster)  [unwired: 1 in, 1 out]
                n258 = property on="Pelletron Voltage (MV):" class="DigNum (strict)"(error in=w489, "Value"=0.005 ("Pelletron Voltage (MV):"), "Caption.Text"="Needle Voltage (MV):") -> (error out=w493:errorcluster)  [unwired: 1 in, 1 out]
              }
              frame False {
                n259 = property on="Constrained Distribution" class="XYGraph (strict)"(error in=w497, "XScale.Minimum"=0.1 ("X Scale.Range:Minimum"), "XScale.Maximum"=200.0 ("X Scale.Range:Maximum")) -> (error out=w496:errorcluster)  [unwired: 1 in, 1 out]
                n260 = property on="Pelletron Voltage (MV):" class="DigNum (strict)"(error in=w496, "Value"=2.17 ("Pelletron Voltage (MV):"), "Caption.Text"="Pelletron Voltage (MV):") -> (error out=w500:errorcluster)  [unwired: 1 in, 1 out]
              }
            }
            n261 = Equal?(x=w455, y="NPL-PC-2" ("x")) -> (x = y?=w450:bool)
            n262 = Equal?(x="Small?", y=w450) -> (x = y?=w447:bool)
            n263 = Select(t=T7."Enabled" ("Disabled"), s=w447, f=T7."Disabled and Grayed Out") -> (s? t:f=w445:T7)
            n264 = property on="Selected Waveforms" class="Arr (strict)"("DisabledEnum"=w445) -> ()  [unwired: 2 in, 2 out]
            n265 = property on="Waveforms" class="Arr (strict)"("DisabledEnum"=w445) -> ()  [unwired: 2 in, 2 out]
            n266 = case shown="True" "Small?" {
              tunnel: w462 -> [w485 w487]
              tunnel: [w484 w486] -> w461
              frame False {
                w483 = FALSE ("If this was the big acc...")
                n267 = property on="If this was the big acc..." class="Bool (strict)"(error in=w485, "Value"=w483, "Visible"=w483) -> (error out=w484:errorcluster)  [unwired: 1 in, 1 out]
              }
              frame True {
                n268 = property on="If this was the big acc..." class="Bool (strict)"(error in=w487, "Visible"=TRUE) -> (error out=w486:errorcluster)  [unwired: 1 in, 1 out]
              }
            }
            n269 = property on="Time Visible" class="DigNum (strict)"("DisabledEnum"=w445) -> ()  [unwired: 2 in, 2 out]
            n270 = property on="Reset Visible Time" class="Bool (strict)"("DisabledEnum"=w445) -> ()  [unwired: 2 in, 2 out]
            n271 = property on="Tab Control" class="TabCtl (strict)"(error in=w461, "Value"=T1."Live Plot" ("Tab Control")) -> (error out=w467:errorcluster)  [unwired: 1 in, 1 out]
            n272 = local read "Small?"() -> (w460:bool)
            n273 = call <userlib>:"last_density_query.vi"("error in (no error)"=w467, "Small?"=w460) -> ("error out"=w469:errorcluster, "Density"=w468:dbl)  [unwired: 8 in]
            n274 = local write "Density (g/cc)"(w468) -> ()
            n275 = call <userlib>:"last_exp_settings_query.vi"("error in (no error)"=w469, "Small?"=w460) -> ("error out"=w470:errorcluster, "Experiment Name"=w472:string, "Group Name"=w471:string)  [unwired: 4 in, 3 out]
            n276 = call <userlib>:"int_to_LV_time.vi"("error in (no error)"=w470) -> ("error out"=w466:errorcluster, "time stamp"=w480:timestamp)  [unwired: 8 in]
            n277 = Build Array(w472) -> (w446:string[])
            n278 = local read "Month"() -> (w481:dbl)
            n279 = local write "Experiment Start"(w480) -> ()
            n280 = Add(x=w481, y=w480) -> (x+y=w477:timestamp)
            n281 = local read "Constraints"() -> (w479:T3)
            n282 = Bundle By Name(cluster=w479, "Upper Timestamp Range"=w477, "Lower Timestamp Range"=w480, "Experiment Group:"=w471, "name array"=w446, "Upper Velocity Limit (km/s)"=299792, "Lower Velocity Limit (km/s)"=w475, "Upper Mass Limit (kg)"=1, "Lower Mass Limit (kg)"=w475, "Experiment Name:"=i32[] [0], "Estimate Quality"=cluster{dbl, dbl} {0.0, 5.0}) -> (w478:T3)
            n283 = local write "Constraints"(w478) -> ()
          }
          event "Waveforms": Mouse Down; "Waveforms": Mouse Up; "Waveforms": Key Up {
            n284 = event-data() -> ()  [unwired: 1 in, 5 out]
            n285 = local read "Selected Waveforms"() -> (w512:u64[])
            n286 = property on="Waveforms" class="Arr (strict)"(error in=w516) -> (error out=w515:errorcluster, "Value"=w513:T4[], "Index Values"=w517:u32[])  [unwired: 1 in, 1 out]
            n287 = Array Size(array=w512) -> (size(s)=w511:i32)
            n288 = call-poly <userlib>:"Empty Array__ogtk.vi"("Array"=w513) -> ("Empty Array?"=w518:bool)  [unwired: 8 in]
            n289 = case shown="False" w518 {
              tunnel: w517 -> [w528 _]
              tunnel: w515 -> [w527 w532]
              tunnel: [w526 w532] -> w514
              tunnel: w513 -> [w525 _]
              tunnel: w511 -> [w524 _]
              tunnel: [w521 _] -> w509
              frame False {
                n290 = Index Array(array=w528) -> (element=w530:u32)  [unwired: 1 in]
                n291 = Decrement(x=w524) -> (x-1=w531:i32)
                n292 = Less?(x=w530, y=w531) -> (x < y?=w529:bool)
                n293 = Array Subset(array=w525, length=w524) -> (w523:T4[])  [unwired: 1 in]
                n294 = Select(t=w530, s=w529, f=w531) -> (s? t:f=w521:u32)
                n295 = Build Array(w521) -> (w522:u32[])
                n296 = property on="Waveforms" class="Arr (strict)"(error in=w527, "Value"=w523, "Index Values"=w522) -> (error out=w526:errorcluster)  [unwired: 1 in, 1 out]
              }
              frame True {
              }
            }
            n297 = call "Filter"() -> ()  [unwired: 10 in, 2 out]
            n298 = property on="Waveform Graph" class="WFGraph (strict)"(error in=w514) -> (error out=w520:errorcluster, "Value"=w508:sgl[][])  [unwired: 1 in, 1 out]
            n299 = local read "Multipliers"() -> (w510:dbl[])
            n300 = Array Size(array=w508) -> (size(s)=w507:i32[])
            n301 = Index Array(array=w510, index=w509) -> (element=w504:dbl)
            n302 = Index Array(array=w507, index=1) -> (element=w505:i32)
            n303 = Multiply(x=w505, y=w504) -> (x*y=w503:dbl)
            n304 = property on="Waveform Graph" class="WFGraph (strict)"(error in=w520, "Val(Sgnl)"=w508, "XScale.Multiplier"=w504) -> (error out=w519:errorcluster)  [unwired: 1 in, 1 out]
            n305 = local write "Max Time"(w503) -> ()
          }
          event "Reset Visible Time": Value Change {
            n306 = event-data() -> ()  [unwired: 1 in, 6 out]
            n307 = property on="Waveform Graph" class="WFGraph (strict)"(error in=w535, "XScale.Minimum"=0.0 ("X Scale.Range:Minimum")) -> (error out=w534:errorcluster)  [unwired: 1 in, 1 out]
            n308 = property on="Max Time" class="DigNum (strict)"(error in=w534) -> (error out=w540:errorcluster, "Value"=w539:dbl)  [unwired: 1 in, 1 out]
            n309 = property on="Time Visible" class="DigNum (strict)"(error in=w540, "Val(Sgnl)"=w539) -> (error out=w538:errorcluster)  [unwired: 1 in, 1 out]
            n310 = property on="Reset Visible Time" class="Bool (strict)"(error in=w538, "Value"=FALSE ("Reset Visible Time")) -> (error out=w537:errorcluster)  [unwired: 1 in, 1 out]
          }
          event "Time Visible": Value Change {
            n311 = event-data() -> ()  [unwired: 1 in, 6 out]
            n312 = property on="Waveform Graph" class="WFGraph (strict)"(error in=w545) -> (error out=w544:errorcluster, "XScale.Minimum"=w543:dbl)  [unwired: 1 in, 1 out]
            n313 = local read "Max Time"() -> (w547:dbl)
            n314 = Add(x=w543, y="Time Visible") -> (x+y=w546:dbl)
            n315 = Less Or Equal?(x=w546, y=w547) -> (x <= y?=w548:bool)
            n316 = case shown="False" w548 {
              tunnel: w547 -> [w549 _]
              tunnel: "Time Visible" -> [w554 _]
              tunnel: w546 -> [_ w557]
              tunnel: w544 -> [w551 w556]
              tunnel: [w553 w555] -> w541
              frame False {
                n317 = property on="Waveform Graph" class="WFGraph (strict)"(error in=w551, "XScale.Maximum"=w549) -> (error out=w550:errorcluster)  [unwired: 1 in, 1 out]
                n318 = Subtract(x=w549, y=w554) -> (x-y=w552:dbl)
                n319 = property on="Waveform Graph" class="WFGraph (strict)"(error in=w550, "XScale.Minimum"=w552) -> (error out=w553:errorcluster)  [unwired: 1 in, 1 out]
              }
              frame True {
                n320 = property on="Waveform Graph" class="WFGraph (strict)"(error in=w556, "XScale.Maximum"=w557) -> (error out=w555:errorcluster)  [unwired: 1 in, 1 out]
              }
            }
          }
          event "Exit": Value Change {
            n321 = event-data() -> ()  [unwired: 1 in, 6 out]
          }
        }
        n322 = case shown="Error" w132 {
          selector: w132 -> [w145 w149]
          tunnel: [w145 w150] -> w131
          tunnel: [w144 w149] -> w130
          frame No Error {
            n323 = case shown="True" "Clear Errors" {
              tunnel: w145 -> [_ w148]
              tunnel: [w147 w148] -> w144
              frame False {
                n324 = local read "error out"() -> (w147:errorcluster)
              }
              frame True {
                n325 = local write "error out"(w148) -> ()
              }
            }
          }
          frame Error {
            n326 = call <vilib>:"Clear Errors.vi"("error in (no error)"=w149) -> ("error out"=w150:errorcluster)  [unwired: 6 in]
            n327 = local write "error out"(w149) -> ()
          }
        }
      }
      n328 = property on="Exit" class="Bool (strict)"(error in=w127, "Value"=FALSE ("Exit")) -> ()  [unwired: 1 in, 2 out]
    }
    frame Error {
    }
  }
  "error out" <- w18
